vi "Cleanup.vi"(8 "error in (no error)":errorcluster, 11 "InfoService in":refnum<class "InfoService.lvclass">) -> (0 "error out":errorcluster)   [LabVIEW 2020, in "Vecto.lvlib" / "InfoService.lvclass"]
uses:
  InfoService.lvclass
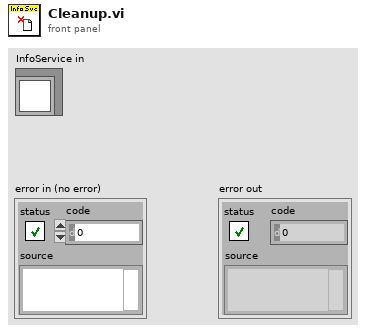
[diagram p1: front panel]
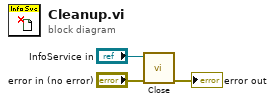
[diagram p0: block diagram]
diagram:
  n1 = call "Close.vi"("error in (no error)"="error in (no error)", "InfoService in"="InfoService in") -> ("error out"=→"error out":errorcluster)  [unwired: 9 in]
